vi "SetParam.vi"(8 "error in (no error)":errorcluster caption="entrée d'erreur (pas d'erreur)", 10 "IterativeImputer":T1={"estimator"="None", "missing_values"="nan", "sample_posterior"=FALSE, "max_iter"=10, "tol"=0.001, "n_nearest_features"=-1, "initial_strategy"="mean", "imputation_order"="ascending", "skip_complete"=FALSE, "min_value"=["None"], "max_value"=["None"], "verbose"=0, "random_state"=-1, "add_indicator"=FALSE} {"random_state" min=-1; "n_nearest_features" min=-1}, 11 "IterativeImputer.lvclass":refnum<class "IterativeImputer.lvclass">) -> (0 "error out":errorcluster caption="sortie d'erreur", 3 "IterativeImputer.lvclass":refnum<class "IterativeImputer.lvclass">)   [LabVIEW 2020, in "IterativeImputer.lvclass"]
doc: "Set Parameters"
uses:
  IterativeImputer.lvclass
  IterativeImputer.lvclass/IterativeImputer.ctl
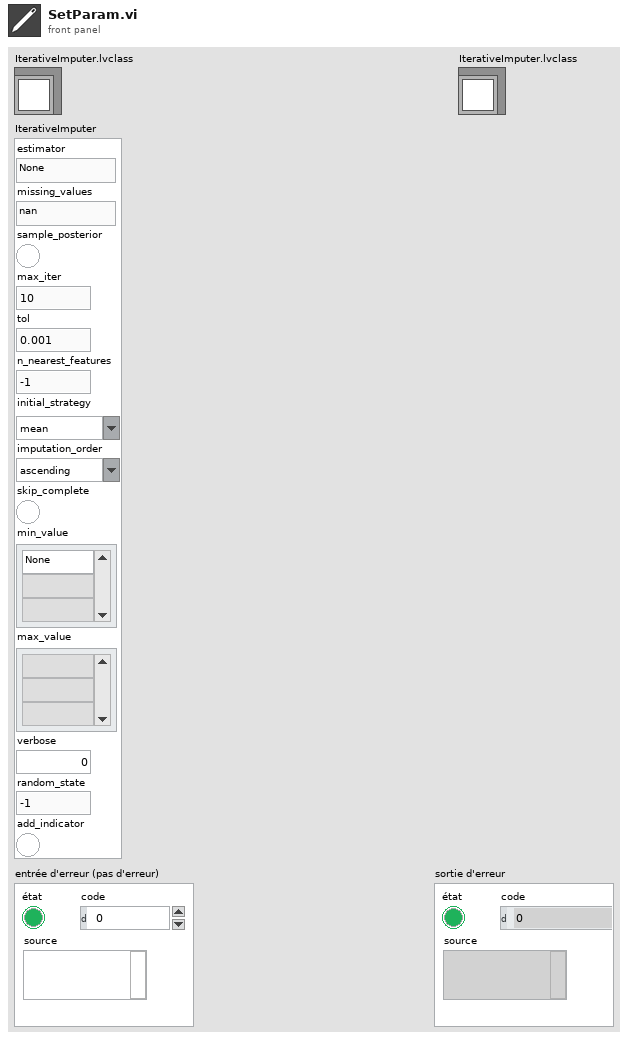
[diagram p1: front panel]
types:
  T1 = cluster{"estimator":string, "missing_values":string, "sample_posterior":bool, "max_iter":i32, "tol":dbl, "n_nearest_features":i32, "initial_strategy":string, "imputation_order":string, "skip_complete":bool, "min_value":string[], "max_value":string[], "verbose":i32, "random_state":i32, "add_indicator":bool}
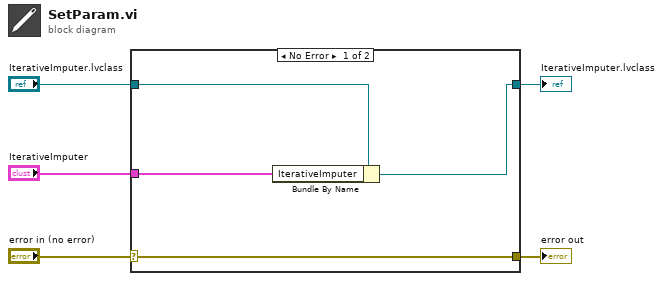
[diagram p0: block diagram]
diagram:
  n1 = case shown="No Error" "error in (no error)" {
    selector: "error in (no error)" -> [w9 w10]
    tunnel: [w9 w10] -> w4
    tunnel: [w7 w11] -> w2
    tunnel: "IterativeImputer.lvclass" -> [w8 w11]
    tunnel: "IterativeImputer" -> [w6 _]
    frame No Error {
      n2 = Bundle By Name(cluster=w8, "IterativeImputer"=w6) -> (w7:refnum<class "IterativeImputer.lvclass">)
    }
    frame Error {
    }
  }
  "error out" <- w4
  "IterativeImputer.lvclass" <- w2
